vi "FlightStatus.vi"() -> ()   [LabVIEW 2010]
uses:
  <vilib>/Utility/miscctls.llb/LV3DPointTypeDef.ctl
  <vilib>/picture/3D Picture Control/NI_3D Picture Control.lvlib
panel:
  out "Battery":dbl format="%.1f"
  out "Flight Mode":bool
  out "Altitude":dbl format="%.1f"
  out "Heading":dbl format="%.1f"
  out "Pitch":dbl format="%.1f"
  out "Roll":dbl format="%.1f"
  out "Motor 8":dbl(slide) scale=1000.0..2000.0
  out "Motor 7":dbl(slide) scale=1000.0..2000.0
  out "Motor 6":dbl(slide) scale=1000.0..2000.0
  out "Motor 5":dbl(slide) scale=1000.0..2000.0
  out "Motor 4":dbl(slide) scale=1000.0..2000.0
  out "Motor 3":dbl(slide) scale=1000.0..2000.0
  out "Motor 2":dbl(slide) scale=1000.0..2000.0
  out "Motor 1":dbl(slide) scale=1000.0..2000.0
  out "Altitude Hold":bool
  out "Motor Status":bool
  out "Aux3":dbl(slide) scale=1000.0..2000.0
  out "Aux2":dbl(slide) scale=1000.0..2000.0
  out "Aux1":dbl(slide) scale=1000.0..2000.0
  out "Mode":dbl(slide) scale=1000.0..2000.0
  out "Right Stick":refnum<vi>(3d-picture)
  out "Left Stick":refnum<vi>(3d-picture)
  out "AI":refnum<vi>(3d-picture)
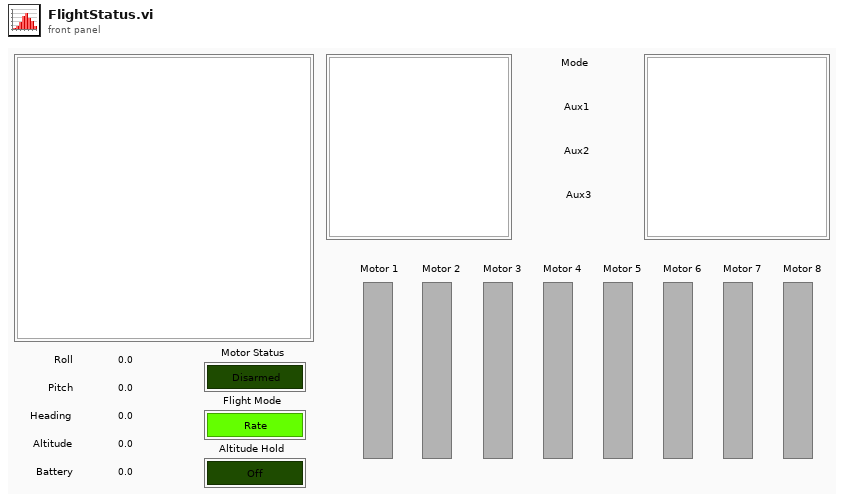
[diagram p1: front panel]
types:
  T1 = cluster{"Error":errorcluster, "PlotNames":string[], "GUIQueue":refnum<queue>, "Telemetry":string, "Format":string, "Equation":string, "IniData":string[][], "Data":dbl[], "RightStick":refnum<vi>, "LeftStick":refnum<vi>, "AH":refnum<vi>, "AHpath":path, "AHposition":refnum<vi>, "AHheading":refnum<vi>, "Receiver":i32, "Motors":i32, "LeftStickScene":refnum<vi>, "RightStickScene":refnum<vi>}
  T2 = enum16{"None", "Spherical", "Flying", "Oriented"}
  T3 = typedef "LV3DPointTypeDef.ctl" = cluster{"X":sgl, "Y":sgl, "Z":sgl}
  T4 = cluster{"Red":sgl, "Green":sgl, "Blue":sgl, "Alpha":sgl}
  T5 = enum8{"Enabled", "Disabled", "Disabled and Grayed Out"}
  T6 = enum32{"invalid app kind", "Development System", "Run Time System", "Student Edition", "Embedded LabVIEW", "Evaluation", "Custom"}
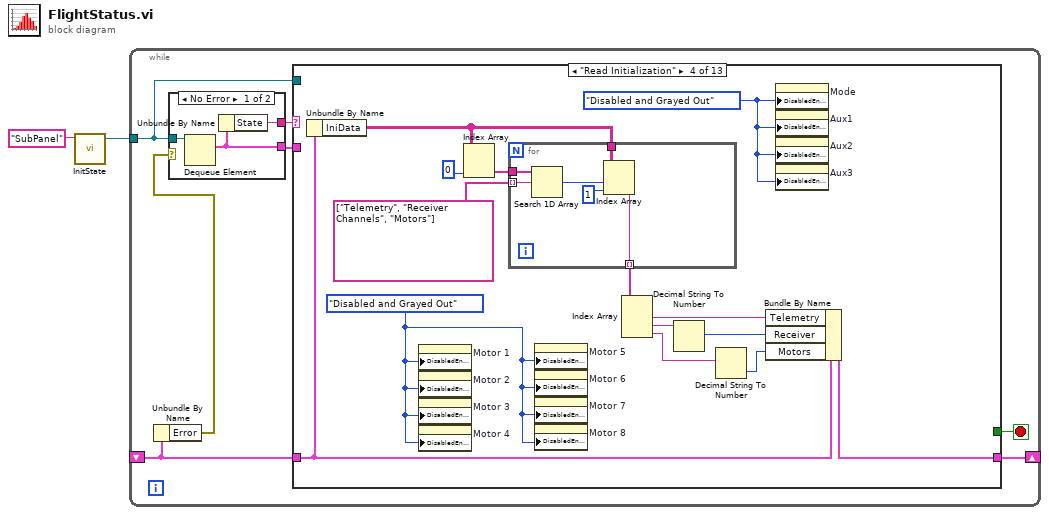
[diagram p0: block diagram]
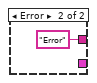
[diagram p2: hidden frame]
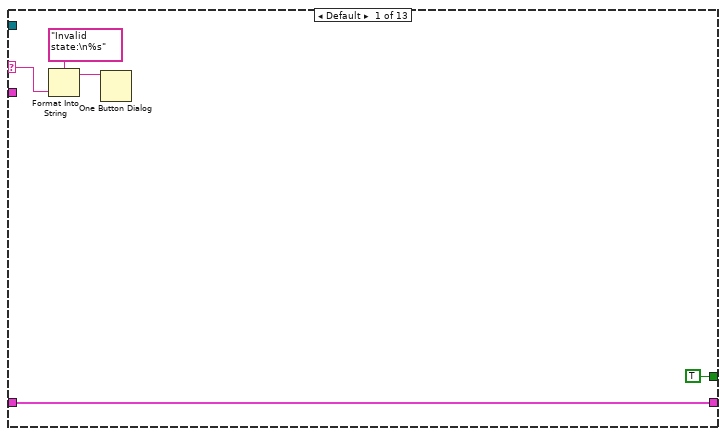
[diagram p3: hidden frame]
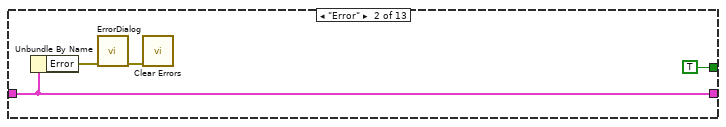
[diagram p4: hidden frame]
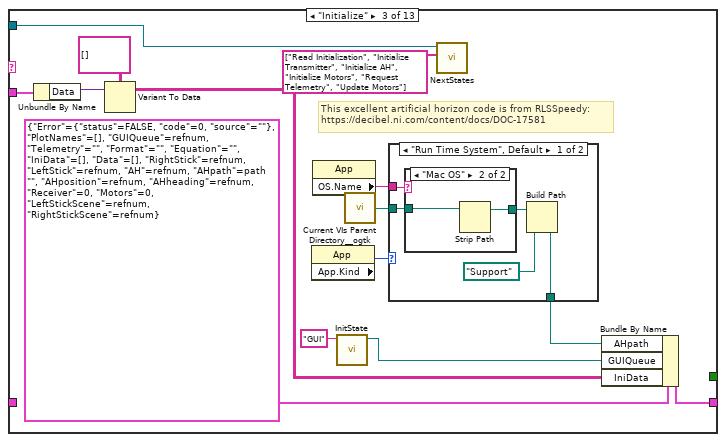
[diagram p5: hidden frame]
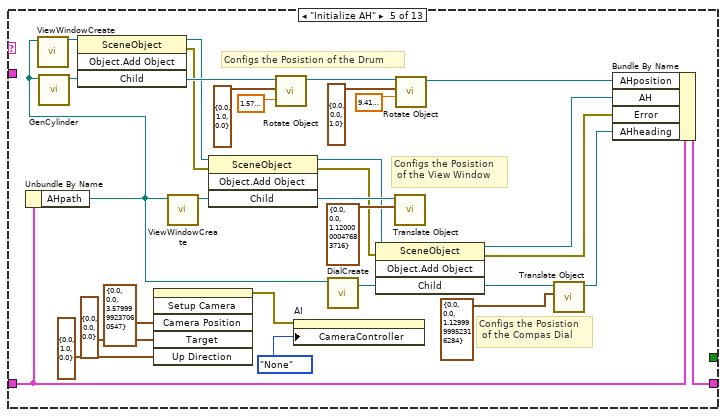
[diagram p8: hidden frame]
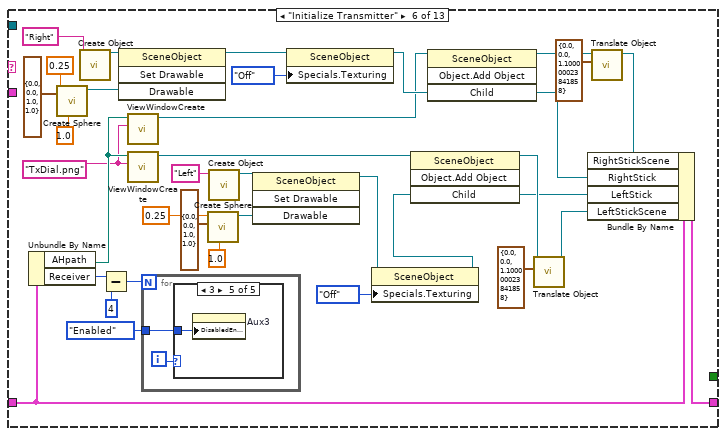
[diagram p9: hidden frame]
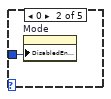
[diagram p11: hidden frame]
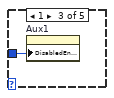
[diagram p12: hidden frame]
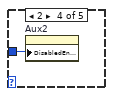
[diagram p13: hidden frame]
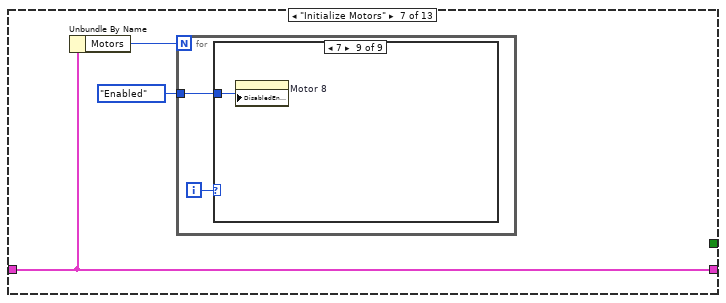
[diagram p14: hidden frame]
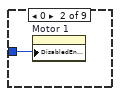
[diagram p16: hidden frame]
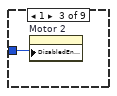
[diagram p17: hidden frame]
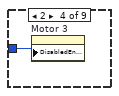
[diagram p18: hidden frame]
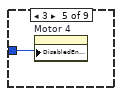
[diagram p19: hidden frame]
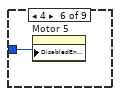
[diagram p20: hidden frame]
diagram:
  n1 = call "InitState.vi"("Name"="SubPanel" ("name (unnamed)")) -> ("Queue Out"=w1:refnum<queue>)  [unwired: 8 in, 1 out]
  n2 = while {
    tunnel: w1 -> [w3]
    shift-right: [w9] -> _
    shift-left: _ -> [w8]
    stop <- w7 stop-if-true
    n3 = Unbundle By Name(w8) -> ("Error"=w6:errorcluster)
    n4 = case shown="No Error" w6 {
      tunnel: [w12 "Error" ("State")] -> w5
      tunnel: [w11 _] -> w4
      tunnel: w3 -> [w10 _]
      frame No Error {
        n5 = Dequeue Element(queue=w10) -> (element=w11:cluster{"State":string, "Data":variant})  [unwired: 2 in, 3 out]
        n6 = Unbundle By Name(w11) -> ("State"=w12:string)
      }
      frame Error {
      }
    }
    n7 = case shown="\"Read Initialization\"" w5 {
      selector: w5 -> [w16 _ _ _ _ _ _ _ _ _ _ _ _]
      tunnel: w4 -> [_ _ w31 _ _ _ _ _ w167 _ _ _ _]
      tunnel: w3 -> [_ _ w27 _ _ _ _ _ w161 _ _ _ _]
      tunnel: [w15 w21 w34 w58 w81 w120 w140 w156 w163 w209 w226 w256 w258] -> w9
      tunnel: w8 -> [w15 w21 _ w59 w82 w119 w140 w158 w164 w209 w226 w256 w258]
      tunnel: [TRUE TRUE _ _ _ _ _ _ _ _ _ _ TRUE] -> w7
      frame Default {
        n8 = Format Into String(format string="Invalid state:\n%s", w16) -> (resulting string=w17:string)  [unwired: 2 in, 1 out]
        n9 = One Button Dialog(message=w17) -> ()  [unwired: 1 in, 1 out]
      }
      frame "Error" {
        n10 = Unbundle By Name(w21) -> ("Error"=w20:errorcluster)
        n11 = call "ErrorDialog.vi"("error in"=w20) -> ("error out"=w19:errorcluster)  [unwired: 10 in]
        n12 = call <vilib>:"Clear Errors.vi"("error in (no error)"=w19) -> ()  [unwired: 6 in, 1 out]
      }
      frame "Initialize" {
        # "This excellent artificial horizon code is from RLSSpeedy:\nhttps://decibel.ni.com/content/docs/DOC-17581"
        n13 = Unbundle By Name(w31) -> ("Data"=w30:variant)
        n14 = Variant To Data(Variant=w30, type=string[][] [] ("subarray")) -> (data=w29:string[][])  [unwired: 1 in, 1 out]
        n15 = property class="App"() -> ("App.Kind"=w26:T6)  [unwired: 2 in, 2 out]
        n16 = property class="App"() -> ("OS.Name"=w24:string)  [unwired: 2 in, 2 out]
        n17 = call "InitState.vi"("Name"="GUI") -> ("Queue Out"=w32:refnum<queue>)  [unwired: 8 in, 1 out]
        n18 = call <userlib>:"Current VIs Parent Directory__ogtk.vi"() -> ("Parent Directory (+ Relative)"=w25:path)  [unwired: 5 in]
        n19 = case shown="\"Run Time System\", Default" w26 {
          tunnel: [w41 w45] -> w23
          tunnel: w25 -> [w39 w45]
          tunnel: w24 -> [w37 _]
          frame "Run Time System", Default {
            n20 = case shown="\"Mac OS\"" w37 {
              tunnel: [w42 w44] -> w40
              tunnel: w39 -> [w42 w43]
              frame Default {
              }
              frame "Mac OS" {
                n21 = Strip Path(path=w43) -> (stripped path=w44:path)  [unwired: 1 out]
              }
            }
            n22 = Build Path(base path=w40, name or relative path=path "Support") -> (appended path=w41:path)
          }
          frame "Development System" {
          }
        }
        n23 = call "NextStates.vi"("States"=string[] ["Read Initialization", "Initialize Transmitter", "Initialize AH", "Initialize Motors", "Request Telemetry", "Update Motors"], "Queue In"=w27) -> ()  [unwired: 8 in, 2 out]
        n24 = Bundle By Name(cluster=T1 {"Error"={"status"=FALSE, "code"=0, "source"=""}, "PlotNames"=[], "GUIQueue"=refnum, "Telemetry"="", "Format"="", "Equation"="", "IniData"=[], "Data"=[], "RightStick"=refnum, "LeftStick"=refnum, "AH"=refnum, "AHpath"=path "", "AHposition"=refnum, "AHheading"=refnum, "Receiver"=0, "Motors"=0, "LeftStickScene"=refnum, "RightStickScene"=refnum}, "AHpath"=w23, "GUIQueue"=w32, "IniData"=w29) -> (w34:T1)
      }
      frame "Read Initialization" {
        w46 = T5."Disabled and Grayed Out" ("Disabled")
        w47 = T5."Disabled and Grayed Out" ("Disabled")
        n25 = Unbundle By Name(w59) -> ("IniData"=w54:string[][])
        n26 = property on="Motor 1" class="Slide (strict)"("DisabledEnum"=w46) -> ()  [unwired: 2 in, 2 out]
        n27 = property on="Motor 2" class="Slide (strict)"("DisabledEnum"=w46) -> ()  [unwired: 2 in, 2 out]
        n28 = property on="Motor 3" class="Slide (strict)"("DisabledEnum"=w46) -> ()  [unwired: 2 in, 2 out]
        n29 = property on="Motor 4" class="Slide (strict)"("DisabledEnum"=w46) -> ()  [unwired: 2 in, 2 out]
        n30 = Index Array(array=w54, index (col)=0 ("index (row)")) -> (element=w56:string[])  [unwired: 1 in]
        n31 = for {
          tunnel: w56 -> [w65]
          tunnel: string[] ["Telemetry", "Receiver Channels", "Motors"] -> [w61] mode=indexing
          tunnel: w54 -> [w64]
          tunnel: [w60] -> w53 mode=indexing
          n32 = Search 1D Array(1D array=w65, element=w61) -> (index of element=w62:i32)  [unwired: 1 in]
          n33 = Index Array(array=w64, index (row)=w62, index (col)=1 ("disabled index (col)")) -> (element=w60:string)
        }
        n34 = property on="Motor 5" class="Slide (strict)"("DisabledEnum"=w46) -> ()  [unwired: 2 in, 2 out]
        n35 = property on="Motor 6" class="Slide (strict)"("DisabledEnum"=w46) -> ()  [unwired: 2 in, 2 out]
        n36 = property on="Motor 7" class="Slide (strict)"("DisabledEnum"=w46) -> ()  [unwired: 2 in, 2 out]
        n37 = property on="Motor 8" class="Slide (strict)"("DisabledEnum"=w46) -> ()  [unwired: 2 in, 2 out]
        n38 = Index Array(array=w53) -> (element #1=w52:string, element #2=w51:string, element #3=w49:string)  [unwired: 3 in]
        n39 = Decimal String To Number(string=w51) -> (number=w50:i32)  [unwired: 2 in, 1 out]
        n40 = Decimal String To Number(string=w49) -> (number=w48:i32)  [unwired: 2 in, 1 out]
        n41 = Bundle By Name(cluster=w59, "Telemetry"=w52, "Receiver"=w50, "Motors"=w48) -> (w58:T1)
        n42 = property on="Mode" class="Slide (strict)"("DisabledEnum"=w47) -> ()  [unwired: 2 in, 2 out]
        n43 = property on="Aux1" class="Slide (strict)"("DisabledEnum"=w47) -> ()  [unwired: 2 in, 2 out]
        n44 = property on="Aux2" class="Slide (strict)"("DisabledEnum"=w47) -> ()  [unwired: 2 in, 2 out]
        n45 = property on="Aux3" class="Slide (strict)"("DisabledEnum"=w47) -> ()  [unwired: 2 in, 2 out]
      }
      frame "Initialize AH" {
        # "Configs the Posistion\n of the Compas Dial"
        # "Configs the Posistion\n of the View Window"
        # "Configs the Posistion of the Drum"
        n46 = Unbundle By Name(w82) -> ("AHpath"=w66:path)
        n47 = call "ViewWindowCreate.vi"("Solid Horizon Path.PNG"=w66) -> ("SceneObject out"=w86:refnum<vi>)  [unwired: 10 in]
        n48 = call "GenCylinder.vi"("Solid Horizon Path.PNG"=w66) -> ("SceneObject out"=w84:refnum<vi>)  [unwired: 10 in]
        n49 = invoke class="SceneObject" method="Object.Add Object"(reference=w86, "Child"=w84) -> (reference out=w87:refnum<vi>, error out=w85:errorcluster, "Child"=w93:refnum<vi>)  [unwired: 2 in, 1 out]
        n50 = invoke on="AI" class="SceneGraphDisp (strict)" method="Setup Camera"("Camera Position"=T3 {"X"=0.0, "Y"=0.0, "Z"=3.58}, "Target"=T3 {"X"=0.0, "Y"=0.0, "Z"=0.0}, "Up Direction"=T3 {"X"=0.0, "Y"=1.0, "Z"=0.0}) -> (error out=w68:errorcluster)  [unwired: 3 in, 5 out]
        n51 = call "ViewWindowCreate.vi"("Solid Horizon Path.PNG"=w66) -> ("SceneObject out"=w83:refnum<vi>)  [unwired: 10 in]
        n52 = invoke class="SceneObject" method="Object.Add Object"(reference=w87, error in=w85, "Child"=w83) -> (reference out=w76:refnum<vi>, error out=w74:errorcluster, "Child"=w88:refnum<vi>)  [unwired: 1 in, 1 out]
        n53 = call <vilib>:"Rotate Object.vi"("Angle"=sgl 1.5799999 ("Angle 2"), "Axis"=cluster{"X":sgl, "Y":sgl, "Z":sgl} {"X"=0.0, "Y"=1.0, "Z"=0.0} ("Axis 2"), "Scene.Object In"=w93) -> ("Scene.Object Out"=w92:refnum<vi>)  [unwired: 7 in, 1 out]
        n54 = property on="AI" class="SceneGraphDisp (strict)"(error in=w68, "CameraController"=T2."None" ("Camera Controller:Type")) -> ()  [unwired: 1 in, 2 out]
        n55 = call "DialCreate.vi"("Solid Horizon Path.PNG"=w66) -> ("SceneObject out"=w77:refnum<vi>)  [unwired: 10 in]
        n56 = invoke class="SceneObject" method="Object.Add Object"(reference=w76, error in=w74, "Child"=w77) -> (reference out=w75:refnum<vi>, error out=w72:errorcluster, "Child"=w78:refnum<vi>)  [unwired: 1 in, 1 out]
        n57 = call <vilib>:"Translate Object.vi"("Translation"=cluster{"X":sgl, "Y":sgl, "Z":sgl} {"X"=0.0, "Y"=0.0, "Z"=1.12} ("Translation 4"), "Scene.Object In"=w88) -> ()  [unwired: 8 in, 2 out]
        n58 = call <vilib>:"Rotate Object.vi"("Angle"=sgl 9.419999 ("Angle 3"), "Axis"=cluster{"X":sgl, "Y":sgl, "Z":sgl} {"X"=0.0, "Y"=0.0, "Z"=1.0} ("Axis 3"), "Scene.Object In"=w92) -> ("Scene.Object Out"=w80:refnum<vi>)  [unwired: 7 in, 1 out]
        n59 = call <vilib>:"Translate Object.vi"("Translation"=cluster{"X":sgl, "Y":sgl, "Z":sgl} {"X"=0.0, "Y"=0.0, "Z"=1.13} ("Translation 5"), "Scene.Object In"=w78) -> ("Scene.Object Out"=w73:refnum<vi>)  [unwired: 8 in, 1 out]
        n60 = Bundle By Name(cluster=w82, "AHposition"=w80, "AH"=w75, "Error"=w72, "AHheading"=w73) -> (w81:T1)
      }
      frame "Initialize Transmitter" {
        w102 = "TxDial.png" ("File")
        n61 = Unbundle By Name(w119) -> ("AHpath"=w103:path, "Receiver"=w118:i32)
        n62 = call <vilib>:"Create Sphere.vi"("Detail"=sgl 1.0, "Color"=T4 {"Red"=0.0, "Green"=0.0, "Blue"=1.0, "Alpha"=1.0}, "Radius"=sgl 0.25) -> ("New Sphere Refnum"=w121:refnum<vi>)  [unwired: 1 in, 7 out]
        n63 = call <vilib>:"Create Object.vi"("Name"="Right") -> ("Scene:New Object"=w125:refnum<vi>)  [unwired: 9 in, 1 out]
        n64 = Subtract(x=w118, y=4) -> (x-y=w116:i32)
        n65 = invoke class="SceneObject" method="Set Drawable"(reference=w125, "Drawable"=w121) -> (reference out=w112:refnum<vi>)  [unwired: 2 in, 3 out]
        n66 = call "ViewWindowCreate.vi"("File"=w102, "Solid Horizon Path.PNG"=w103) -> ("SceneObject out"=w104:refnum<vi>)  [unwired: 9 in]
        n67 = call "ViewWindowCreate.vi"("File"=w102, "Solid Horizon Path.PNG"=w103) -> ("SceneObject out"=w101:refnum<vi>)  [unwired: 9 in]
        n68 = for {
          N: w116 -> [_]
          tunnel: T5."Enabled" ("Disabled") -> [w132]
          i -> [w133]
          n69 = case shown="3" w133 {
            tunnel: w132 -> [_ w134 w135 w136 w137]
            frame Default {
            }
            frame 0 {
              n70 = property on="Mode" class="Slide (strict)"("DisabledEnum"=w134) -> ()  [unwired: 2 in, 2 out]
            }
            frame 1 {
              n71 = property on="Aux1" class="Slide (strict)"("DisabledEnum"=w135) -> ()  [unwired: 2 in, 2 out]
            }
            frame 2 {
              n72 = property on="Aux2" class="Slide (strict)"("DisabledEnum"=w136) -> ()  [unwired: 2 in, 2 out]
            }
            frame 3 {
              n73 = property on="Aux3" class="Slide (strict)"("DisabledEnum"=w137) -> ()  [unwired: 2 in, 2 out]
            }
          }
        }
        n74 = call <vilib>:"Create Sphere.vi"("Detail"=sgl 1.0, "Color"=T4 {"Red"=0.0, "Green"=0.0, "Blue"=1.0, "Alpha"=1.0}, "Radius"=sgl 0.25) -> ("New Sphere Refnum"=w124:refnum<vi>)  [unwired: 1 in, 7 out]
        n75 = call <vilib>:"Create Object.vi"("Name"="Left") -> ("Scene:New Object"=w128:refnum<vi>)  [unwired: 9 in, 1 out]
        n76 = invoke class="SceneObject" method="Set Drawable"(reference=w128, "Drawable"=w124) -> (reference out=w105:refnum<vi>)  [unwired: 2 in, 3 out]
        n77 = property class="SceneObject"(reference=w112, "Specials.Texturing"=enum16{"Inherit Value", "Off", "On"}."Off" ("Specials:Texturing")) -> (reference out=w111:refnum<vi>)  [unwired: 1 in, 1 out]
        n78 = property class="SceneObject"(reference=w105, "Specials.Texturing"=enum16{"Inherit Value", "Off", "On"}."Off" ("Specials:Texturing")) -> (reference out=w100:refnum<vi>)  [unwired: 1 in, 1 out]
        n79 = invoke class="SceneObject" method="Object.Add Object"(reference=w101, "Child"=w100) -> (reference out=w98:refnum<vi>, "Child"=w96:refnum<vi>)  [unwired: 2 in, 2 out]
        n80 = invoke class="SceneObject" method="Object.Add Object"(reference=w104, "Child"=w111) -> (reference out=w110:refnum<vi>, "Child"=w114:refnum<vi>)  [unwired: 2 in, 2 out]
        n81 = call <vilib>:"Translate Object.vi"("Translation"=cluster{"X":sgl, "Y":sgl, "Z":sgl} {"X"=0.0, "Y"=0.0, "Z"=1.1}, "Scene.Object In"=w98) -> ("Scene.Object Out"=w97:refnum<vi>)  [unwired: 8 in, 1 out]
        n82 = call <vilib>:"Translate Object.vi"("Translation"=cluster{"X":sgl, "Y":sgl, "Z":sgl} {"X"=0.0, "Y"=0.0, "Z"=1.1}, "Scene.Object In"=w110) -> ("Scene.Object Out"=w107:refnum<vi>)  [unwired: 8 in, 1 out]
        n83 = Bundle By Name(cluster=w119, "RightStickScene"=w107, "RightStick"=w114, "LeftStick"=w96, "LeftStickScene"=w97) -> (w120:T1)
      }
      frame "Initialize Motors" {
        n84 = Unbundle By Name(w140) -> ("Motors"=w139:i32)
        n85 = for {
          N: w139 -> [_]
          tunnel: T5."Enabled" ("Disabled") -> [w141]
          i -> [w142]
          n86 = case shown="7" w142 {
            tunnel: w141 -> [_ w143 w144 w145 w146 w147 w148 w149 w150]
            frame Default {
            }
            frame 0 {
              n87 = property on="Motor 1" class="Slide (strict)"("DisabledEnum"=w143) -> ()  [unwired: 2 in, 2 out]
            }
            frame 1 {
              n88 = property on="Motor 2" class="Slide (strict)"("DisabledEnum"=w144) -> ()  [unwired: 2 in, 2 out]
            }
            frame 2 {
              n89 = property on="Motor 3" class="Slide (strict)"("DisabledEnum"=w145) -> ()  [unwired: 2 in, 2 out]
            }
            frame 3 {
              n90 = property on="Motor 4" class="Slide (strict)"("DisabledEnum"=w146) -> ()  [unwired: 2 in, 2 out]
            }
            frame 4 {
              n91 = property on="Motor 5" class="Slide (strict)"("DisabledEnum"=w147) -> ()  [unwired: 2 in, 2 out]
            }
            frame 5 {
              n92 = property on="Motor 6" class="Slide (strict)"("DisabledEnum"=w148) -> ()  [unwired: 2 in, 2 out]
            }
            frame 6 {
              n93 = property on="Motor 7" class="Slide (strict)"("DisabledEnum"=w149) -> ()  [unwired: 2 in, 2 out]
            }
            frame 7 {
              n94 = property on="Motor 8" class="Slide (strict)"("DisabledEnum"=w150) -> ()  [unwired: 2 in, 2 out]
            }
          }
        }
      }
      frame "Request Telemetry" {
        n95 = Unbundle By Name(w158) -> ("GUIQueue"=w154:refnum<queue>, "Telemetry"=w153:string)
        n96 = call "NextState.vi"("Data"=w153, "State"="Request Telemetry", "Queue In"=w154) -> ("Error Out"=w151:errorcluster, "Queue Out"=w152:refnum<queue>)  [unwired: 7 in]
        n97 = call "NextState.vi"("Error In"=w151, "State"="Read Continuous", "Queue In"=w152) -> ("Error Out"=w157:errorcluster)  [unwired: 7 in, 1 out]
        n98 = Bundle By Name(cluster=w158, "Error"=w157) -> (w156:T1)
      }
      frame "Update" {
        n99 = Unbundle By Name(w167) -> ("Data"=w166:variant)
        n100 = Variant To Data(Variant=w166, type=dbl[][] []) -> (data=w165:dbl[][])  [unwired: 1 in, 1 out]
        n101 = Index Array(array=w165) -> (element=w162:dbl[])  [unwired: 2 in]
        n102 = Bundle By Name(cluster=w164, "Data"=w162) -> (w163:T1)
        n103 = call "NextStates.vi"("States"=string[] ["Update AH", "Update Transmitter", "Update Motors"], "Queue In"=w161) -> ()  [unwired: 8 in, 2 out]
      }
      frame "Update AH" {
        # "Roll Transform"
        # "Pitch Transform"
        # "Resets the Roll for \nthe Pitch transform"
        n104 = Unbundle By Name(w209) -> ("AHposition"=w181:refnum<vi>, "AHheading"=w180:refnum<vi>, "Data"=w187:dbl[])  [unwired: 1 out]
        n105 = Index Array(array=w187) -> (element #1=w178:dbl, element #2=w177:dbl, element #3=w176:dbl, element #4=w175:dbl, element #5=→"Altitude":dbl, element #6=w173:dbl)  [unwired: 6 in]
        n106 = Equal?(x=1.0, y=w178) -> (x = y?=→"Motor Status":bool)
        n107 = Equal?(x=w173, y=1.0 ("x")) -> (x = y?=→"Altitude Hold":bool)
        n108 = expression code="x * 57.2957795"(w177) -> (w171:dbl)
        "Roll" <- w171
        n109 = expression code="x * 57.2957795"(w176) -> (w182:dbl)
        "Pitch" <- w182
        n110 = expression code="x * 57.2957795"(w175) -> (w179:dbl)
        "Heading" <- w179
        n111 = feedback #1(0.0 ("New Roll Value")) -> (w201:dbl)
        n112 = call "RollCalc.vi"("Previous Roll Value"=w201, "Roll Input"=0.0) -> ("New Roll Value"=w191:dbl, "Adjustment to be Made"=w202:dbl)  [unwired: 8 in]
        n113 = call <vilib>:"Rotate Object.vi"("Angle"=w202, "Axis"=cluster{"X":sgl, "Y":sgl, "Z":sgl} {"X"=0.0, "Y"=0.0, "Z"=1.0} ("Axis 2"), "Scene.Object In"=w181) -> ("Scene.Object Out"=w198:refnum<vi>)  [unwired: 7 in, 1 out]
        n114 = Negate(x=w171) -> (-x=w170:dbl)
        n115 = Negate(x=w182) -> (-x=w172:dbl)
        n116 = feedback #2(0.0 ("New Roll Value")) -> (w195:dbl)
        n117 = call "PitchCalc.vi"("Previous Pitch Value"=w195, "Pitch Control"=w172) -> ("New Pitch Value"=w197:dbl, "Adjustment to be made"=w196:dbl)  [unwired: 8 in]
        n118 = feedback-in #2(w197) -> ()
        n119 = Negate(x=w179) -> (-x=w169:dbl)
        n120 = call <vilib>:"Rotate Object.vi"("Angle"=w196, "Axis"=cluster{"X":sgl, "Y":sgl, "Z":sgl} {"X"=1.0, "Y"=0.0, "Z"=0.0} ("Axis 2"), "Scene.Object In"=w198) -> ("Scene.Object Out"=w192:refnum<vi>)  [unwired: 7 in, 1 out]
        n121 = feedback #3(0.0 ("New Roll Value")) -> (w185:dbl)
        n122 = call "RollCalc.vi"("Previous Roll Value"=w185, "Roll Input"=w169) -> ("New Roll Value"=w183:dbl, "Adjustment to be Made"=w184:dbl)  [unwired: 8 in]
        n123 = feedback-in #3(w183) -> ()
        n124 = call "RollCalc.vi"("Previous Roll Value"=w191, "Roll Input"=w170) -> ("New Roll Value"=w189:dbl, "Adjustment to be Made"=w190:dbl)  [unwired: 8 in]
        n125 = feedback-in #1(w189) -> ()
        n126 = call <vilib>:"Rotate Object.vi"("Angle"=w184, "Axis"=cluster{"X":sgl, "Y":sgl, "Z":sgl} {"X"=0.0, "Y"=0.0, "Z"=1.0} ("Axis 2"), "Scene.Object In"=w180) -> ()  [unwired: 7 in, 2 out]
        n127 = call <vilib>:"Rotate Object.vi"("Angle"=w190, "Axis"=cluster{"X":sgl, "Y":sgl, "Z":sgl} {"X"=0.0, "Y"=0.0, "Z"=1.0} ("Axis 2"), "Scene.Object In"=w192) -> ()  [unwired: 7 in, 2 out]
      }
      frame "Update Transmitter" {
        n128 = Unbundle By Name(w226) -> ("LeftStick"=w227:refnum<vi>, "RightStick"=w228:refnum<vi>, "Data"=w225:dbl[])
        n129 = Index Array(array=w225, index #1=8 ("index"), index #2=9 ("index"), index #3=6 ("index"), index #4=7 ("index"), index #5=10 ("index"), index #6=11 ("index")) -> (element #1=w210:dbl, element #2=w222:dbl, element #3=w221:dbl, element #4=w220:dbl, element #5=→"Mode":dbl, element #6=→"Aux1":dbl, element #7=→"Aux2":dbl, element #8=→"Aux3":dbl)  [unwired: 2 in]
        n130 = expression code="(0.002*x) - 3"(w210) -> (w211:dbl)
        n131 = expression code="(0.002*x) - 3"(w222) -> (w239:dbl)
        n132 = expression code="(0.002*x) - 3"(w221) -> (w233:dbl)
        n133 = expression code="(0.002*x) - 3"(w220) -> (w234:dbl)
        n134 = call <vilib>:"Clear Transformation.vi"("Object Refnum In"=w228) -> ("error out"=w229:errorcluster, "Object Refnum Out"=w230:refnum<vi>)  [unwired: 9 in]
        n135 = call <vilib>:"Clear Transformation.vi"("Object Refnum In"=w227) -> ("error out"=w235:errorcluster, "Object Refnum Out"=w236:refnum<vi>)  [unwired: 9 in]
        n136 = Bundle By Name(cluster=cluster{"X":sgl, "Y":sgl, "Z":sgl} {"X"=0.0, "Y"=0.0, "Z"=0.0} ("Translation"), "X"=w233, "Y"=w234) -> (w232:cluster{"X":sgl, "Y":sgl, "Z":sgl})
        n137 = Bundle By Name(cluster=cluster{"X":sgl, "Y":sgl, "Z":sgl} {"X"=0.0, "Y"=0.0, "Z"=0.0} ("Translation"), "X"=w211, "Y"=w239) -> (w238:cluster{"X":sgl, "Y":sgl, "Z":sgl})
        n138 = call <vilib>:"Translate Object.vi"("error in (no error)"=w229, "Translation"=w232, "Scene.Object In"=w230) -> ()  [unwired: 7 in, 2 out]
        n139 = call <vilib>:"Translate Object.vi"("error in (no error)"=w235, "Translation"=w238, "Scene.Object In"=w236) -> ()  [unwired: 7 in, 2 out]
      }
      frame "Update Motors" {
        n140 = Unbundle By Name(w256) -> ("LeftStickScene"=→"Left Stick":refnum<vi>, "RightStickScene"=→"Right Stick":refnum<vi>, "AH"=→"AI":refnum<vi>, "Data"=w255:dbl[])
        n141 = Index Array(array=w255, index #1=14 ("index")) -> (element #1=→"Motor 1":dbl, element #2=→"Motor 2":dbl, element #3=→"Motor 3":dbl, element #4=→"Motor 4":dbl, element #5=→"Motor 5":dbl, element #6=→"Motor 6":dbl, element #7=→"Motor 7":dbl, element #8=→"Motor 8":dbl, element #9=→"Battery":dbl, element #10=w240:dbl)  [unwired: 9 in]
        n142 = Not Equal To 0?(x=w240) -> (x != 0?=→"Flight Mode":bool)
      }
      frame "Shutdown" {
      }
    }
  }
